vi "VSSGoToAngle.vi"(10 "orientation":dbl format="%#_13g", 11 "dest_orientation":dbl) -> (2 "AngleError":dbl, 3 "v_ang":dbl, 5 "Invert?":bool)   [LabVIEW 2021]
panel:
  in  "Limits":cluster{"output high":dbl, "output low":dbl}={"output high"=100.0, "output low"=-100.0}
  in  "PID gains in":T1={"proportional gain (Kc)"=1.8, "integral time (Ti, min)"=0.0, "derivative time (Td, min)"=2.5}
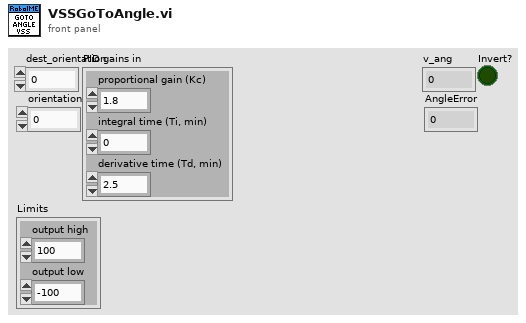
[diagram p1: front panel]
types:
  T1 = cluster{"proportional gain (Kc)":dbl, "integral time (Ti, min)":dbl, "derivative time (Td, min)":dbl}
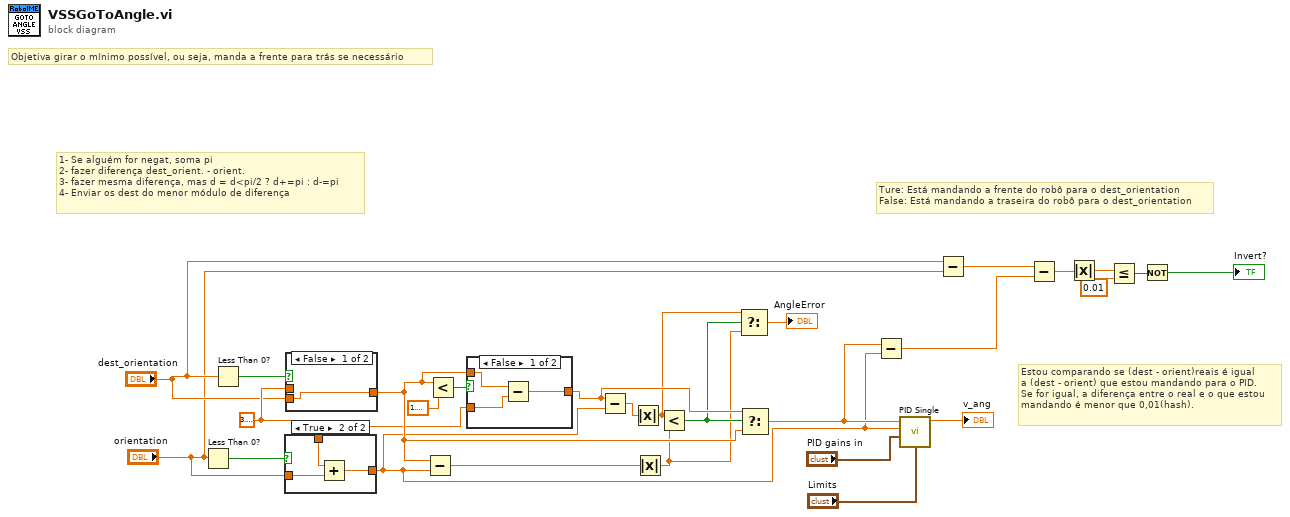
[diagram p0: block diagram]
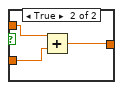
[diagram p2: hidden frame]
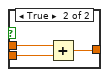
[diagram p4: hidden frame]
diagram:
  w16 = 3.141592653589793
  # "Estou comparando se (dest - orient)reais é igual \na (dest - orient) que estou mandando para o PID.\nSe for igual, a diferença entre o real e o que estou\nmandando é menor que 0,01(hash)."
  # "Ture: Está mandando a frente do robô para o dest_orientation\nFalse: Está mandando a traseira do robô para o dest_orientation"
  # "Objetiva girar o mínimo possível, ou seja, manda a frente para trás se necessário"
  # "1- Se alguém for negat, soma pi\n2- fazer diferença dest_orient. - orient.\n3- fazer mesma diferença, mas d = d<pi/2 ? d+=pi : d-=pi\n4- Enviar os dest do menor módulo de diferença"
  n1 = Less Than 0?(x="orientation") -> (x < 0?=w24:bool)
  n2 = Less Than 0?(x="dest_orientation") -> (x < 0?=w23:bool)
  n3 = case shown="True" w24 {
    tunnel: "orientation" -> [w28 w31]
    tunnel: [w28 w30] -> w8
    tunnel: w16 -> [_ w29]
    frame False {
    }
    frame True {
      n4 = Add(x=w29, y=w31) -> (x+y=w30:dbl)
    }
  }
  n5 = case shown="False" w23 {
    tunnel: "dest_orientation" -> [w32 w35]
    tunnel: [w32 w34] -> w17
    tunnel: w16 -> [_ w33]
    frame False {
    }
    frame True {
      n6 = Add(x=w33, y=w35) -> (x+y=w34:dbl)
    }
  }
  n7 = Subtract(x=w17, y=w8) -> (x-y=w19:dbl)
  n8 = Less?(x=w17, y=1.5707963267948966) -> (x < y?=w21:bool)
  n9 = case shown="False" w21 {
    tunnel: w16 -> [w37 w41]
    tunnel: w17 -> [w38 w40]
    tunnel: [w36 w39] -> w18
    frame False {
      n10 = Subtract(x=w38, y=w37) -> (x-y=w36:dbl)
    }
    frame True {
      n11 = Add(x=w40, y=w41) -> (x+y=w39:dbl)
    }
  }
  n12 = Subtract(x=w18, y=w8) -> (x-y=w20:dbl)
  n13 = Absolute Value(x=w20) -> (abs(x)=w14:dbl)
  n14 = Absolute Value(x=w19) -> (abs(x)=w13:dbl)
  n15 = Less?(x=w14, y=w13) -> (x < y?=w15:bool)
  n16 = Select(t=w14, s=w15, f=w13) -> (s? t:f=→"AngleError":dbl)
  n17 = Select(t=w18, s=w15, f=w17) -> (s? t:f=w9:dbl)
  n18 = Subtract(x=w9, y=w8) -> (x-y=w6:dbl)
  n19 = call "PID Single.vi"("Limits"="Limits", "PID gains in"="PID gains in", "Variable"=w8, "Setpoint"=w9) -> ("Out"=→"v_ang":dbl)  [unwired: 7 in]
  n20 = Subtract(x="dest_orientation", y="orientation") -> (x-y=w7:dbl)
  n21 = Subtract(x=w7, y=w6) -> (x-y=w5:dbl)
  n22 = Absolute Value(x=w5) -> (abs(x)=w4:dbl)
  n23 = Less Or Equal?(x=w4, y=0.01) -> (x <= y?=w2:bool)
  n24 = Not(x=w2) -> (.not. x?=→"Invert?":bool)
